vi "SDA - Analise e calibracao - COM CALC DE FREQ.vi"() -> ()   [LabVIEW 2019]
uses:
  <vilib>/Utility/file.llb/Read From Spreadsheet File (DBL).vi
  <vilib>/Utility/file.llb/Read Delimited Spreadsheet (DBL).vi
  <vilib>/Analysis/NI_AALPro.lvlib
  <vilib>/gmath/NI_Gmath.lvlib
  <vilib>/measure/NI_MABase.lvlib
panel:
  out "ROCOF deviation 2":dbl[](graph)
  in  "F/s":dbl=25.0 format="%#_13g"
  in  "upper":dbl=5.0 format="%#_13g"
  in  "bottom":dbl format="%#_13g"
  in  "bottom":i32=2
  in  "upper":i32=100
  in  "bottom":i32=2
  in  "upper":i32=50
  in  "K (%)":dbl=100.0 format="%#_13g"
  in  "bottom":i32=-180
  in  "upper":i32=180
  in  "upper":i32=65
  in  "bottom":i32=55
  in  "Amplitude base":dbl=1.25 format="%#_13g"
  in  "p.u. ?":bool=TRUE
  in  "Numeric":dbl
  out "output cluster":cluster{i32, i32}
  in  "offset":dbl format="%0.2p"
  in  "phase":dbl format="%.2p"
  in  "amplitude":dbl=1.0 format="%0.2p"
  in  "frequency":dbl=10.0 format="%0.2p"
  out "delay time":dbl format="%#_6f"
  in  "y":dbl
  out "fractional index or x":dbl format="%#_7g"
  in  "threshold y":dbl=0.95
  out "spread value":dbl
  out "lenght":i32
  in  "kept interval":i32=25
  out "Table 2":string[][](table)
  in  "Labels Size":u32=24
  in  "X label":T1(ring)=enum."medidas"
  in  "Tab Control":T2(tab)
  in  "Tab Control 2":T3(tab)
  out "Magnitude absolute deviation":dbl[](graph)
  out "Absolute phase deviation":dbl[](graph)
  out "Magnitude deviation":dbl[](graph)
  out "Phase deviation":dbl[](graph)
  out "Phase":dbl[][](graph)
  out "Magnitude":dbl[][](graph)
  out "TVE":dbl[](graph)
  in  "Tab Control 3":T3(tab)
  out "Absolute freq. deviation":dbl[](graph)
  out "Absolute ROCOF deviation":dbl[](graph)
  out "Frequency deviation":dbl[](graph)
  out "ROCOF deviation":dbl[](graph)
  out "Frequency":dbl[][](graph)
  out "ROCOF":dbl[][](graph)
  out "Frequency deviation 2":dbl[](graph)
  out "Curve fit":dbl[][](graph)
  out "ROCOF\nreference":dbl[](array[numeric])
  out "ROCOF\nmeasured":dbl[](array[numeric])
  out "Frequency\nmeasured":dbl[](array[numeric])
  out "Frequency\nreference":dbl[](array[numeric])
  out "Phase\nmeasured":dbl[](array[numeric])
  out "Phase\nreference":dbl[](array[numeric])
  out "Magnitude\nmeasured":dbl[](array[numeric])
  out "Magnitude\nreference":dbl[](array[numeric])
  in  "polynomial order":i32=2
  in  "Type":T4(ring)=enum."Linear"
  out "Coefficients":string[][](table) caption="Table"
  in  "X data":T5(ring)
  in  "Y data":T5(ring)=enum."Magnitude deviation"
  out "Fit deviation":dbl[](graph)
  out "Correlation\ncoefficient (R)":dbl format="%.7g"
  out "R^2":dbl format="%.7g"
  in  "busca freq":dbl
  out "XY Graph 3":cluster{dbl[], dbl[]}(graph)
  out "XY Graph 2":cluster{dbl[], dbl[]}(graph)
  out "fractional index":dbl format="%_6g"
  out "x*y":dbl
  in  "fractional index or x 3":dbl
  out "ângulo corresp":dbl
  out "mag correspondente":dbl
  in  "frequency 2":dbl
  out "TVE Histogram":T6(graph)
  out "Frequency Error Histogram":T6(graph)
  out "Magnitude Error Histogram":T6(graph)
  out "Phase Error Histogram":T6(graph)
  in  "final":i32
  in  "Interval":bool
  in  "index":i32
  out "nº de amostras":i32
  in  "del interval":i32=25
  in  "Exclude\ninterval":bool
  in  "Archive name":path=path "D:/Resultados/teste.txt"
  # "Fase x freq"
  # "Mag. x mag."
  # "Synchrophasors Data Analysis"
  # "Main Errors"
  # "Max"
  # "Mean"
  # "Min"
  # "Magnitude (%)"
  # "Phase (º)"
  # "TVE (%)"
  # "Freq. (Hz)"
  # "ROCOF (Hz/s)"
  # "Amplitude"
  # "Frequency"
  # "Phase"
  # "Harmonic"
  # "Freq. Interf."
  # "Modulation\nFrequency"
  # "Time"
  # "(frames/second)"
  # "Tamanho para dissertação:\n312x732"
  # "EXTRA"
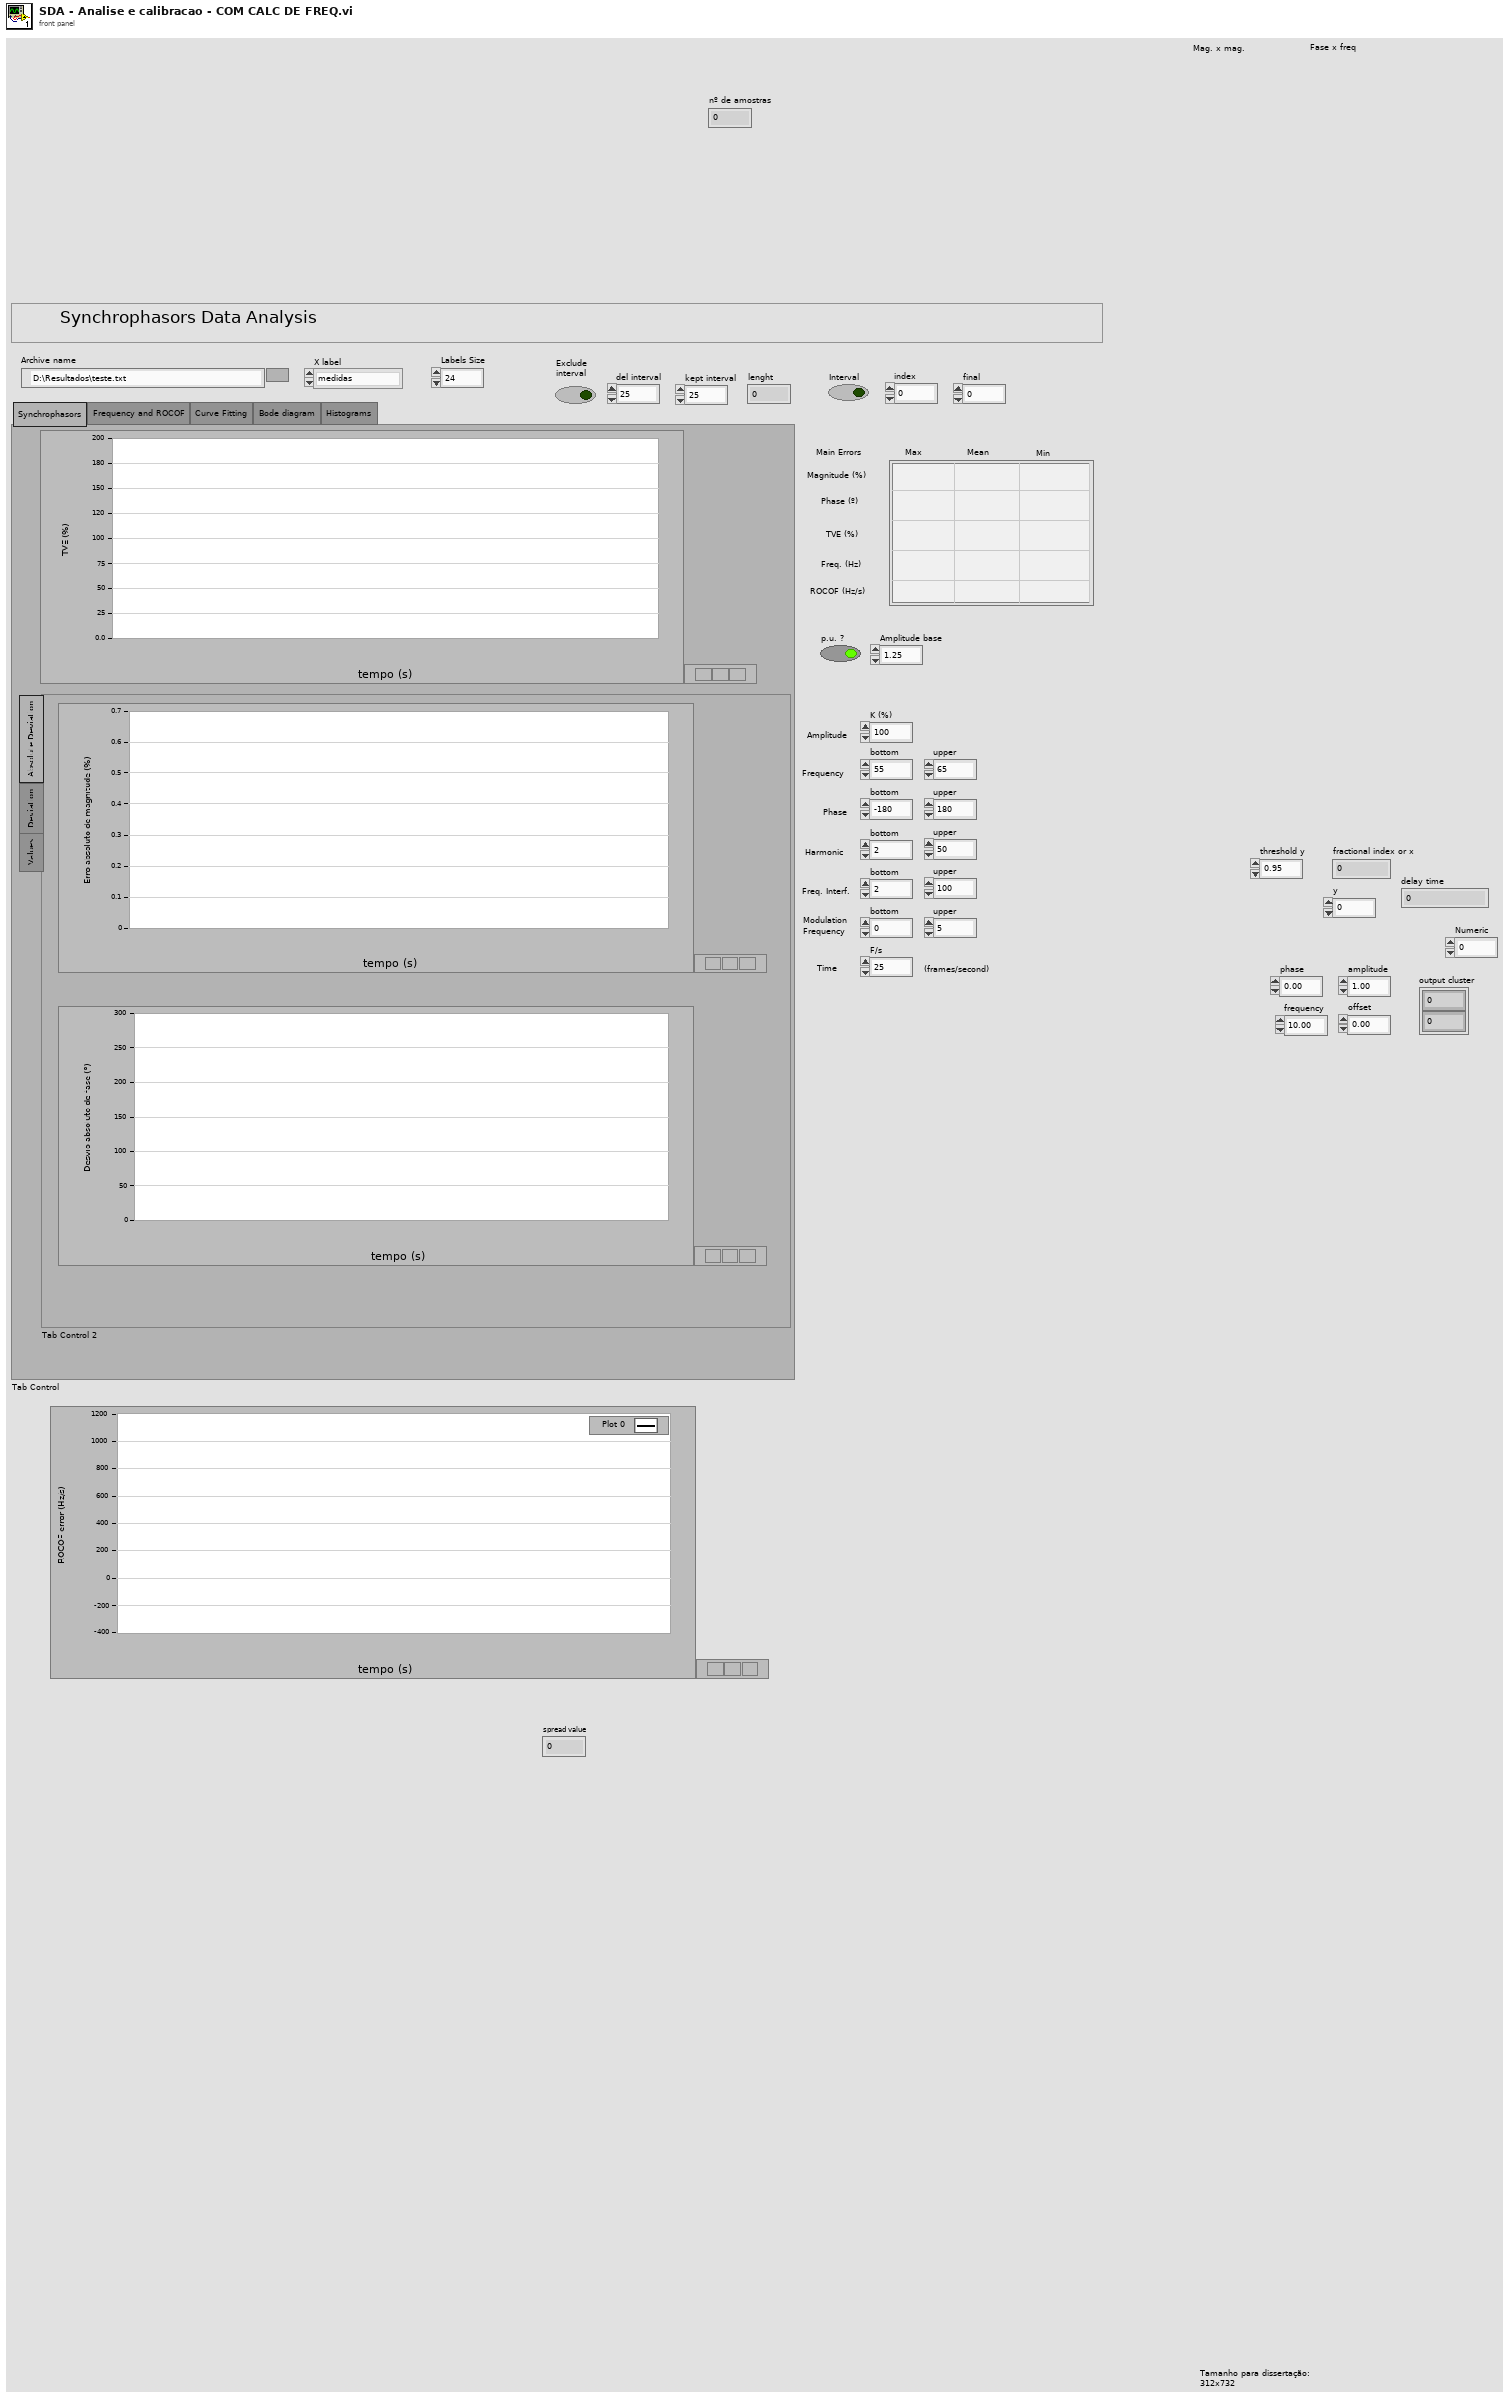
[diagram p1: front panel]
types:
  T1 = enum16{"tempo (s)", "medidas", "Amplitude (%)", "Ângulo (°)", "Frequência (Hz)", "ROCOF (Hz/s)", "Harmônica (.ª)", "Frequência de interferência (Hz)", "Frequência de modulação (Hz)"}
  T2 = enum32{"Synchrophasors", "Frequency and ROCOF", "Curve Fitting", "Bode diagram", "Histograms"}
  T3 = enum32{"Absolute Deviation", "Deviation", "Values"}
  T4 = enum16{"Exponencial", "Logarithm", "Linear", "Polynomial", "Sinusoidal"}
  T5 = enum16{"Magnitude reference", "Magnitude measured", "Magnitude deviation", "Phase reference", "Phase measured", "Phase deviation", "Frequency reference", "Frequency measured", "Frequency deviation"}
  T6 = cluster{"X Values":dbl[], "Histogram: h(x)":i32[]}
  T7 = cluster{"max ref":dbl, "min ref":dbl, "mean ref":dbl, "max dev":dbl, "min dev":dbl, "mean dev":dbl, "max meas":dbl, "min meas":dbl, "mean meas":dbl}
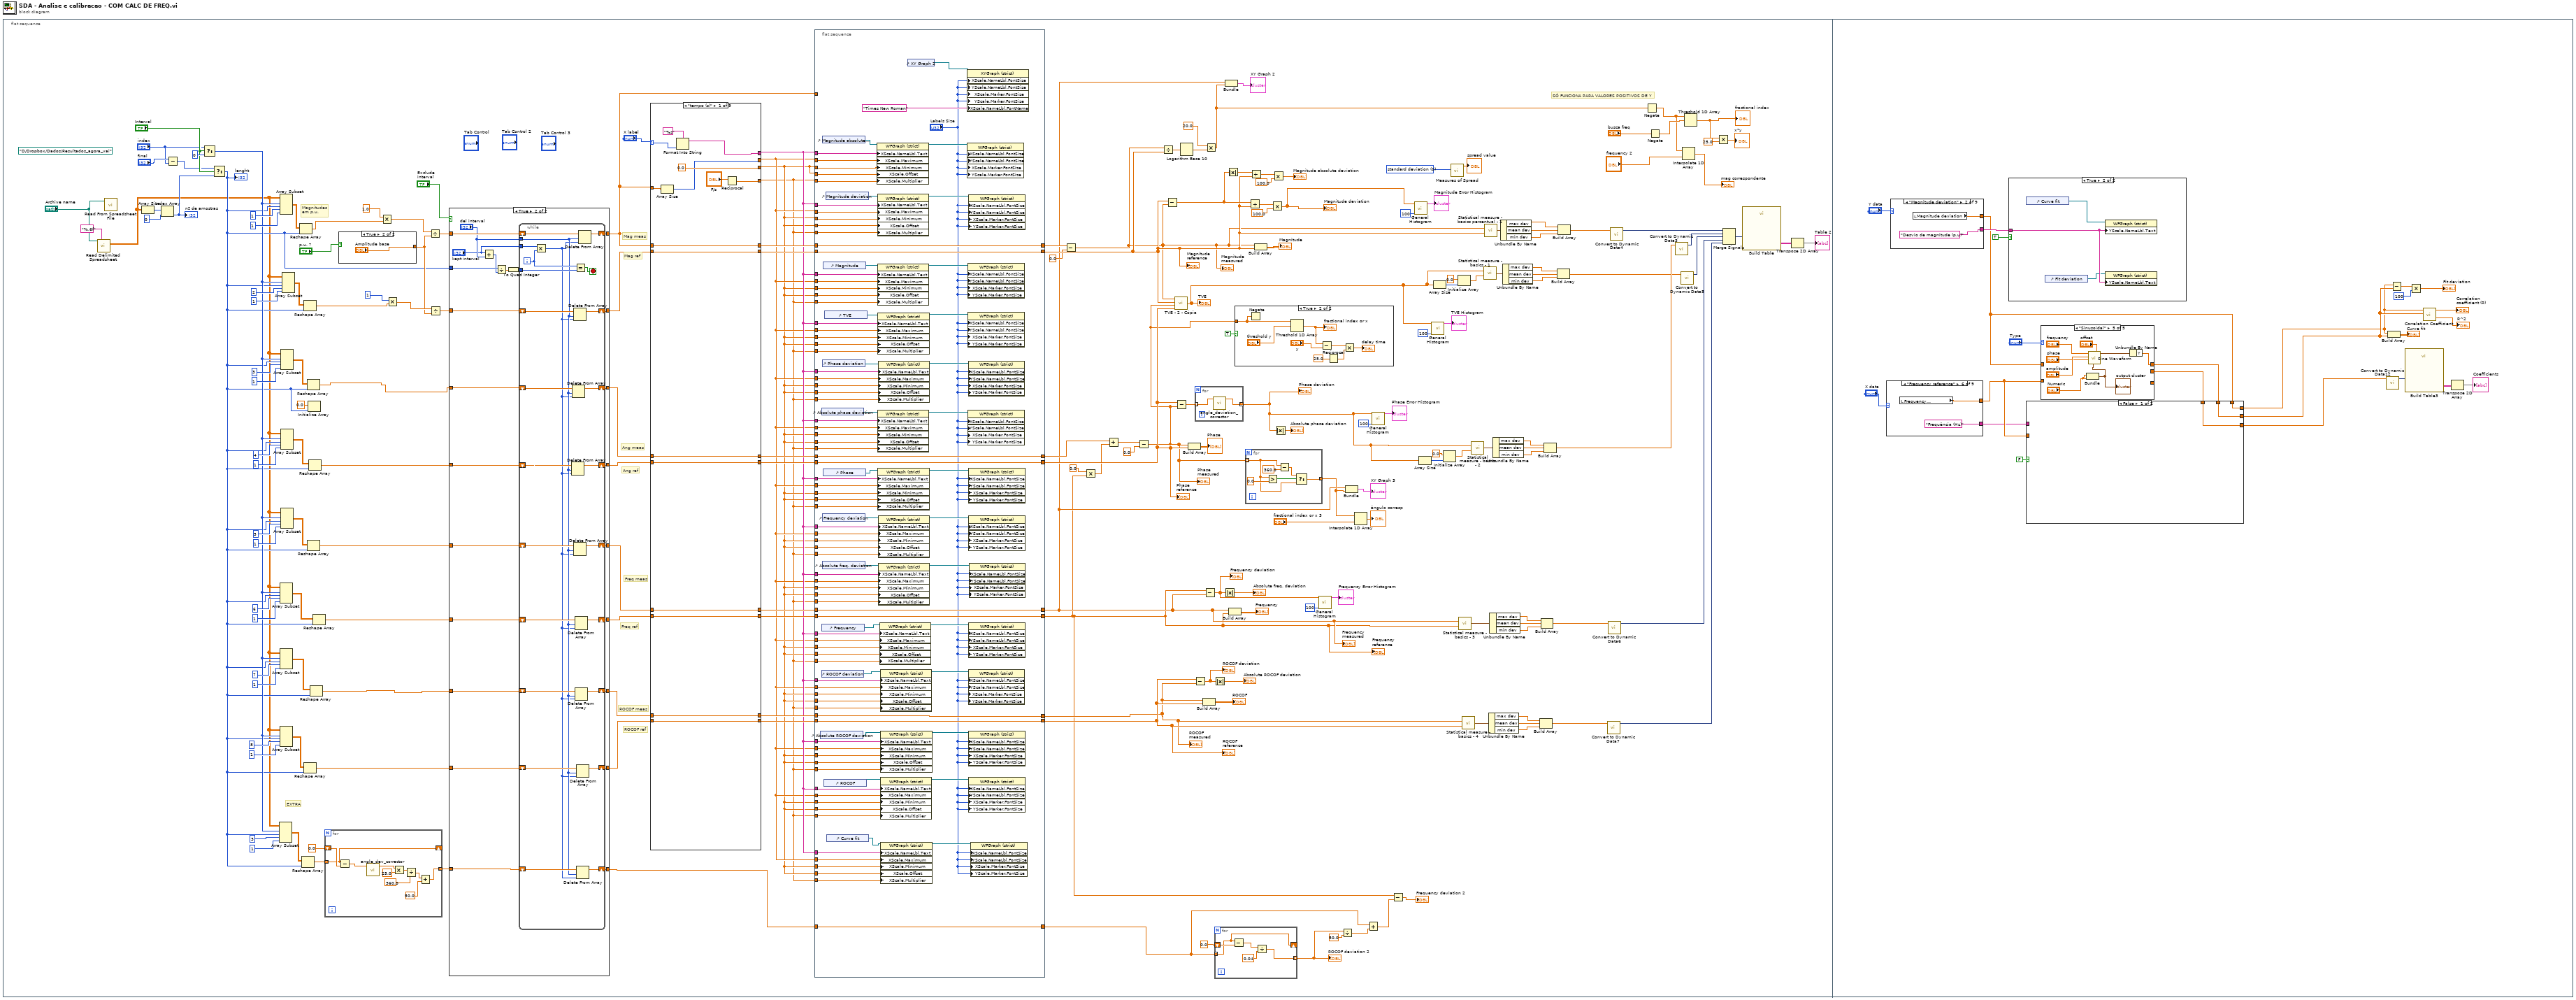
[diagram p0: block diagram]
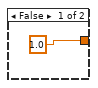
[diagram p3: hidden frame]
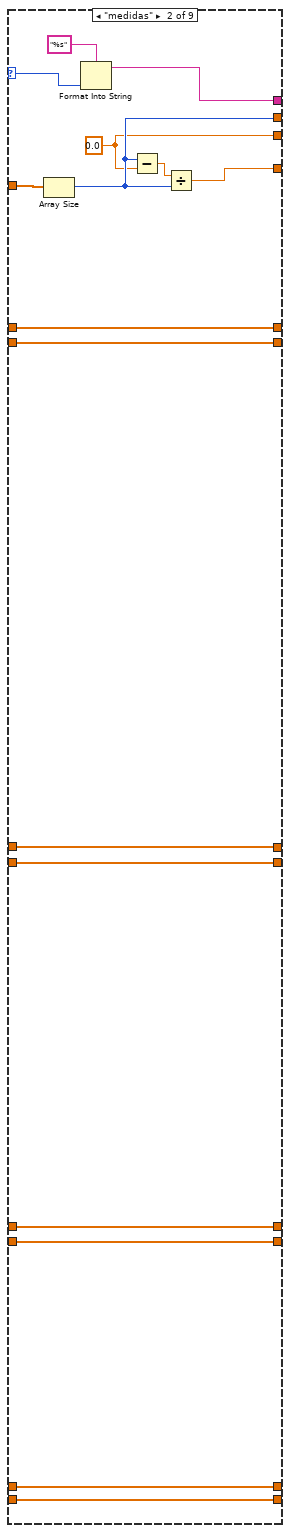
[diagram p4: hidden frame]
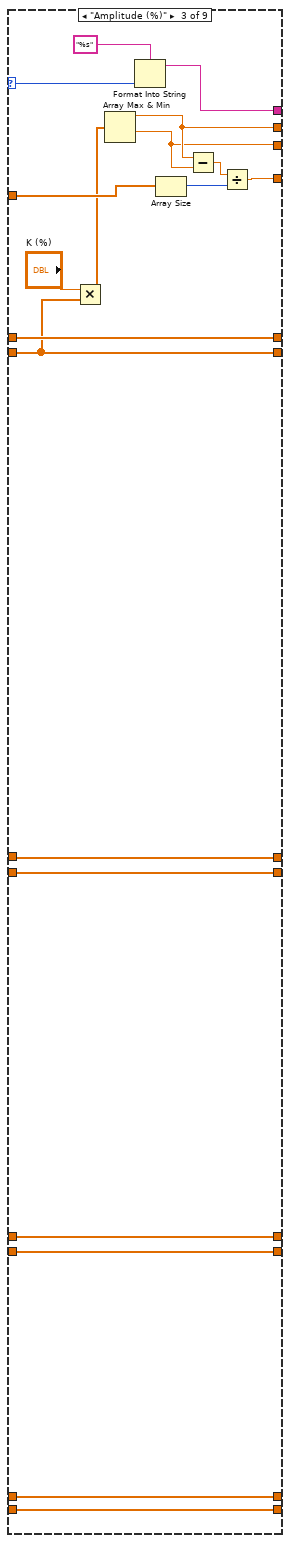
[diagram p5: hidden frame]
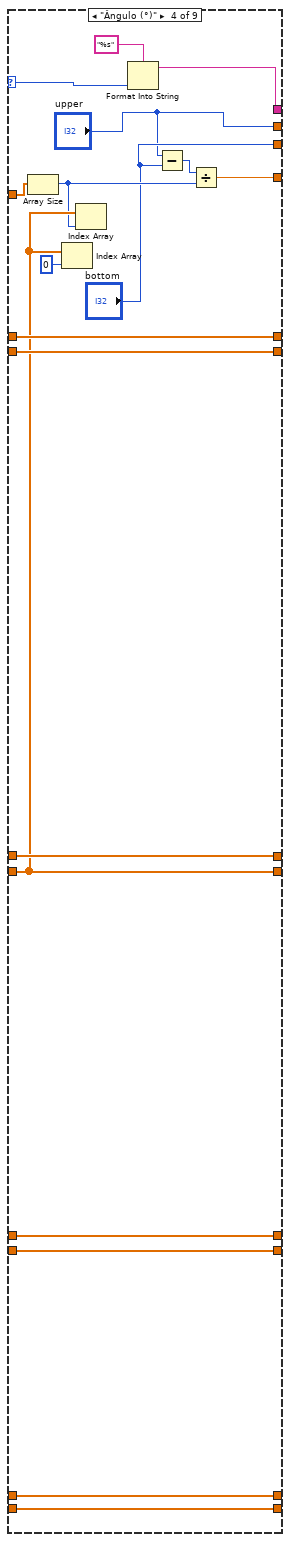
[diagram p6: hidden frame]
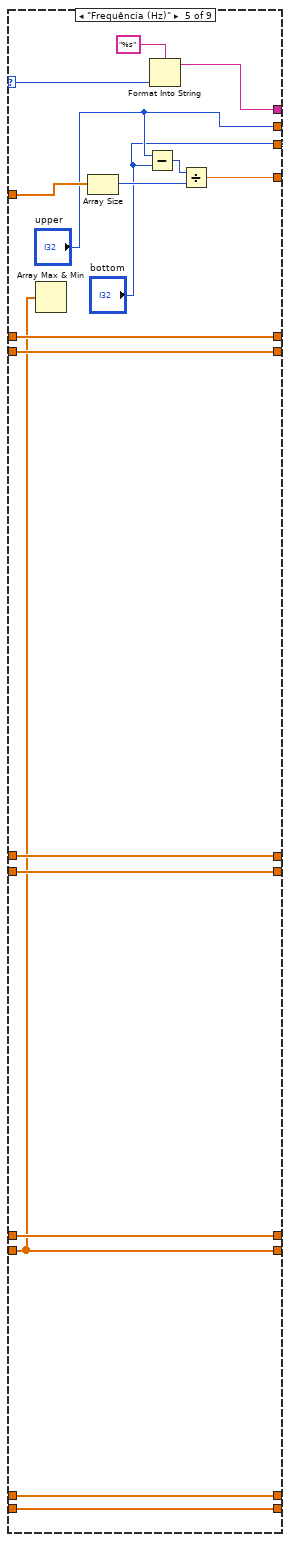
[diagram p7: hidden frame]
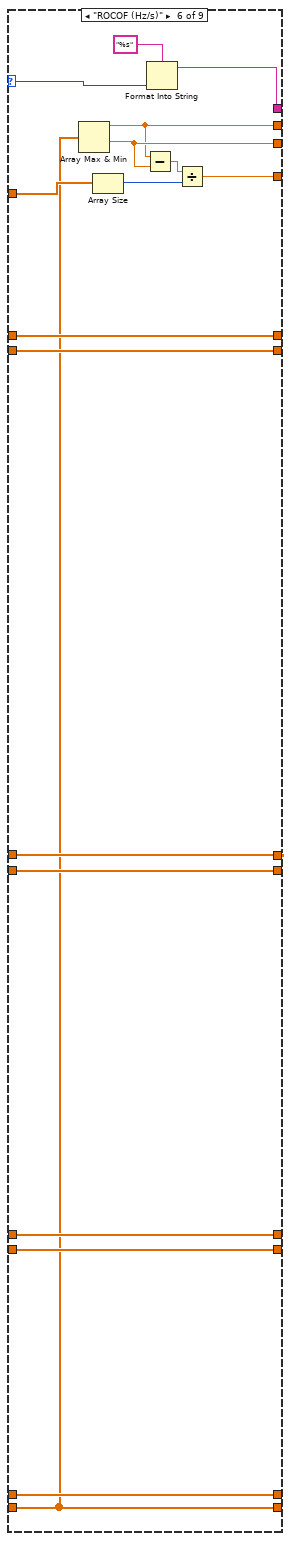
[diagram p8: hidden frame]
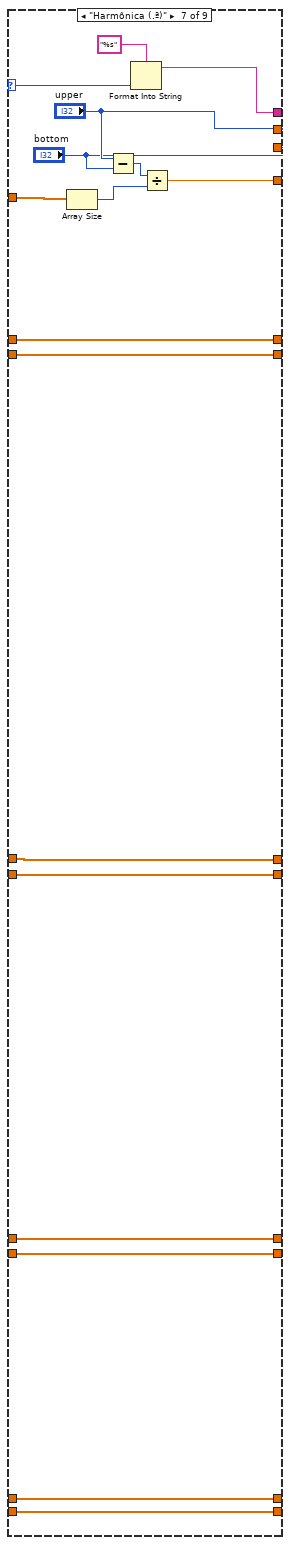
[diagram p9: hidden frame]
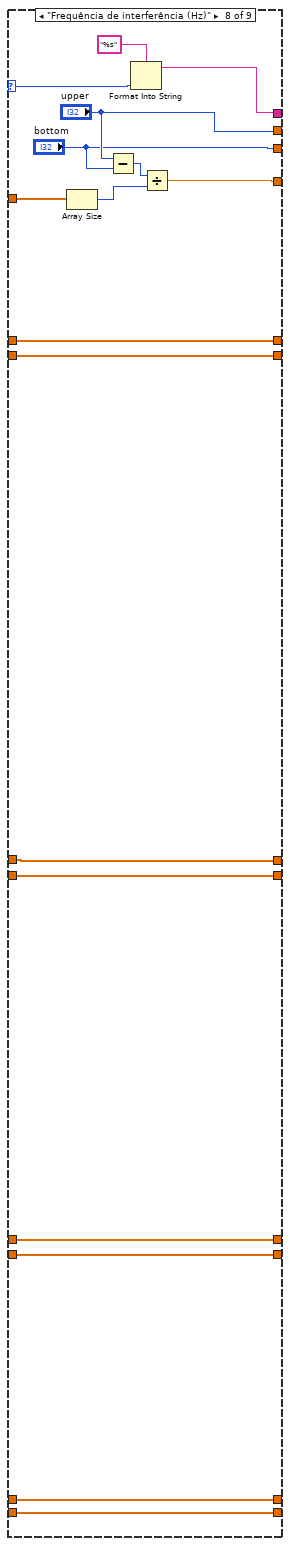
[diagram p10: hidden frame]
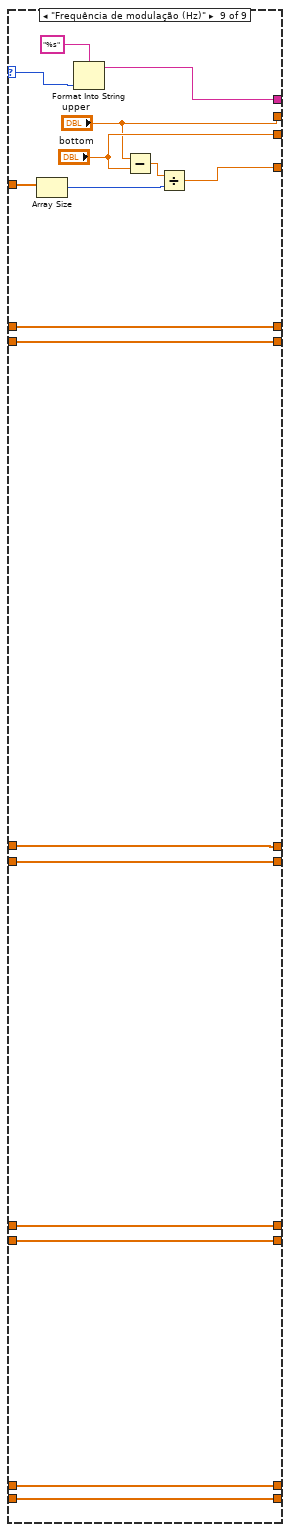
[diagram p11: hidden frame]
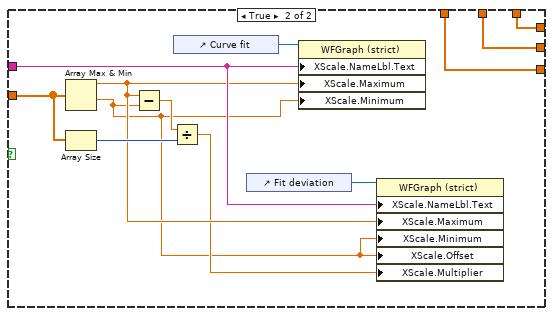
[diagram p13: hidden frame]
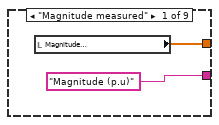
[diagram p15: hidden frame]
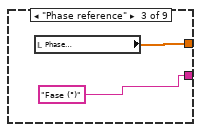
[diagram p16: hidden frame]
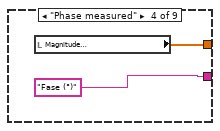
[diagram p17: hidden frame]
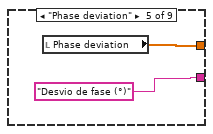
[diagram p18: hidden frame]
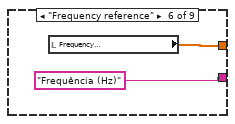
[diagram p19: hidden frame]
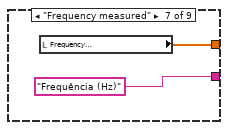
[diagram p20: hidden frame]
diagram:
  n1 = flat-sequence {
    frame #0 {
      w77 = 0 items=["standard deviation", "range", "mean absolute deviation", "interquartile range"] ("type")
      (unwired) path "D:/Dropbox/Dados/Resultados_agora_vai" ("file path (use dialog)")
      # "EXTRA"
      # "SÓ FUNCIONA PARA VALORES POSITIVOS DE Y"
      # "Magnitudes\nem p.u."
      # "ROCOF ref"
      # "ROCOF meas"
      # "Freq ref"
      # "Freq meas"
      # "Ang ref"
      # "Ang meas"
      # "Mag meas"
      # "Mag ref"
      n2 = call-poly <vilib>:"Read Delimited Spreadsheet.vi"("file path (dialog if empty)"="Archive name", "format (%.3f)"="%.6f") -> ("all rows"=w13:dbl[][])  [unwired: 8 in, 5 out]
      n3 = call-poly <vilib>:"Read From Spreadsheet File.vi"("file path (dialog if empty)"="Archive name") -> ()  [unwired: 6 in, 5 out]
      n4 = Array Size(array=w13) -> (size(s)=w189:i32[])
      n5 = Index Array(array=w189, index=0) -> (element=w121:i32)
      "nº de amostras" <- w121
      n6 = Subtract(x="final", y="index") -> (x-y=w124:i32)
      n7 = Select(t="index", s="Interval", f=0) -> (s? t:f=w17:i32)
      n8 = Select(t=w124, s="Interval", f=w121) -> (s? t:f=w16:i32)
      "lenght" <- w16
      n9 = Array Subset(array=w13, index (row)=w17, length (row)=w16, index (col)=3 ("index"), length (col)=1 ("length")) -> (w18:dbl[][])
      n10 = Array Subset(array=w13, index (row)=w17, length (row)=w16, index (col)=1 ("index"), length (col)=1 ("length")) -> (w190:dbl[][])
      n11 = Array Subset(array=w13, index (row)=w17, length (row)=w16, index (col)=6 ("index"), length (col)=1 ("length")) -> (w173:dbl[][])
      n12 = Array Subset(array=w13, index (row)=w17, length (row)=w16, index (col)=7 ("index"), length (col)=1 ("length")) -> (w170:dbl[][])
      n13 = Array Subset(array=w13, index (row)=w17, length (row)=w16, index (col)=8 ("index"), length (col)=1 ("length")) -> (w91:dbl[][])
      n14 = Array Subset(array=w13, index (row)=w17, length (row)=w16, index (col)=4 ("index"), length (col)=1 ("length")) -> (w179:dbl[][])
      n15 = Array Subset(array=w13, index (row)=w17, length (row)=w16, index (col)=5 ("index"), length (col)=1 ("length")) -> (w176:dbl[][])
      n16 = Array Subset(array=w13, index (row)=w17, length (row)=w16, index (col)=3 ("index"), length (col)=1 ("length")) -> (w182:dbl[][])
      n17 = Array Subset(array=w13, index (row)=w17, length (row)=w16, index (col)=2 ("index"), length (col)=1 ("length")) -> (w185:dbl[][])
      n18 = Reshape Array(w190, w16) -> (w69:dbl[])
      n19 = Reshape Array(w18, w16) -> (w8:dbl[])
      n20 = Reshape Array(w185, w16) -> (w67:dbl[])
      n21 = Reshape Array(w91, w16) -> (w90:dbl[])
      n22 = Reshape Array(w182, w16) -> (w39:dbl[])
      n23 = Reshape Array(w176, w16) -> (w142:dbl[])
      n24 = Initialize Array(0.0 ("element"), w16) -> ()  [unwired: 1 out]
      n25 = Reshape Array(w179, w16) -> (w141:dbl[])
      n26 = Reshape Array(w170, w16) -> (w23:dbl[])
      n27 = Reshape Array(w173, w16) -> (w143:dbl[])
      n28 = for {
        tunnel: w8 -> [w203] mode=indexing
        shift-right: [w203] -> _
        shift-left: 0.0 -> [w207]
        tunnel: [w201] -> w10 mode=indexing
        n29 = Subtract(x=w203, y=w207) -> (x-y=w199:dbl)
        n30 = call "angle_dev_corrector.vi"("angle"=w199) -> ("angle corrected"=w198:dbl)  [unwired: 6 in, 2 out]
        n31 = Multiply(x=w198, y=25.0) -> (x*y=w205:dbl)
        n32 = Divide(x=w205, y=360.0) -> (x/y=w200:dbl)
        n33 = Add(x=w200, y=50.0) -> (x+y=w201:dbl)
      }
      n34 = case shown="True" "p.u. ?" {
        tunnel: [1.0 "Amplitude base"] -> w22
        frame False {
        }
        frame True {
        }
      }
      n35 = Multiply(x=1.0, y=w69) -> (x*y=w68:dbl[])
      n36 = Multiply(x=1, y=w67) -> (x*y=w66:dbl[])
      n37 = Divide(x=w68, y=w22) -> (x/y=w101:dbl[])
      n38 = Divide(x=w66, y=w22) -> (x/y=w100:dbl[])
      n39 = case shown="True" "Exclude\ninterval" {
        tunnel: w101 -> [w498 w522]
        tunnel: [w498 w521] -> w58
        tunnel: w90 -> [w491 w517]
        tunnel: w23 -> [w492 w503]
        tunnel: w143 -> [w493 w514]
        tunnel: w142 -> [w494 w512]
        tunnel: w141 -> [w495 w510]
        tunnel: w39 -> [w496 w518]
        tunnel: w100 -> [w497 w520]
        tunnel: [w497 w519] -> w119
        tunnel: [w496 w508] -> w117
        tunnel: [w495 w509] -> w118
        tunnel: [w494 w511] -> w116
        tunnel: [w493 w513] -> w115
        tunnel: [w492 w515] -> w113
        tunnel: [w491 w516] -> w114
        tunnel: w16 -> [_ w507]
        tunnel: w10 -> [w490 w500]
        tunnel: [w490 w499] -> w9
        frame False {
        }
        frame True {
          n40 = Add(x="kept interval", y="del interval") -> (x+y=w505:i32)
          n41 = Divide(x=w507, y=w505) -> (x/y=w502:dbl)
          n42 = To Quad Integer(1:w502) -> (0:w501:i64)
          n43 = while {
            tunnel: "del interval" -> [w525]
            shift-right: [w544] -> w521
            shift-left: w522 -> [w545]
            shift-right: [w543] -> w519
            shift-left: w520 -> [w542]
            shift-right: [w540] -> w508
            shift-left: w518 -> [w541]
            shift-right: [w538] -> w509
            shift-left: w510 -> [w539]
            shift-right: [w536] -> w511
            shift-left: w512 -> [w537]
            shift-right: [w534] -> w513
            shift-left: w514 -> [w535]
            shift-right: [w532] -> w515
            shift-left: w503 -> [w533]
            shift-right: [w530] -> w516
            shift-left: w517 -> [w531]
            tunnel: w501 -> [w529]
            tunnel: "kept interval" -> [w527]
            shift-right: [w523] -> w499
            shift-left: w500 -> [w526]
            i -> [w528]
            stop <- w546 stop-if-true
            n44 = Multiply(x=w527, y=w528) -> (x*y=w524:i32)
            n45 = Delete From Array(array=w539, length=w525, index=w524) -> (array with subset deleted=w538:dbl[])  [unwired: 1 out]
            n46 = Delete From Array(array=w541, length=w525, index=w524) -> (array with subset deleted=w540:dbl[])  [unwired: 1 out]
            n47 = Delete From Array(array=w542, length=w525, index=w524) -> (array with subset deleted=w543:dbl[])  [unwired: 1 out]
            n48 = Delete From Array(array=w537, length=w525, index=w524) -> (array with subset deleted=w536:dbl[])  [unwired: 1 out]
            n49 = Equal?(x=w528, y=w529) -> (x = y?=w546:bool)
            n50 = Delete From Array(array=w535, length=w525, index=w524) -> (array with subset deleted=w534:dbl[])  [unwired: 1 out]
            n51 = Delete From Array(array=w533, length=w525, index=w524) -> (array with subset deleted=w532:dbl[])  [unwired: 1 out]
            n52 = Delete From Array(array=w531, length=w525, index=w524) -> (array with subset deleted=w530:dbl[])  [unwired: 1 out]
            n53 = Delete From Array(array=w526, length=w525, index=w524) -> (array with subset deleted=w523:dbl[])  [unwired: 1 out]
            n54 = Delete From Array(array=w545, length=w525, index=w524) -> (array with subset deleted=w544:dbl[])  [unwired: 1 out]
          }
        }
      }
      n55 = case shown="\"tempo (s)\"" "X label" {
        selector: "X label" -> [w341 w356 w375 w395 w411 w429 w454 w463 w482]
        tunnel: w58 -> [w342 w357 w386 w394 w412 w430 w451 w460 w483]
        tunnel: w119 -> [w350 w366 w372 w403 w409 w427 w448 w471 w485]
        tunnel: [w350 w366 w372 w403 w409 w427 w448 w471 w485] -> w103
        tunnel: w58 -> [w351 w367 w383 w404 w421 w428 w449 w472 w486]
        tunnel: [w351 w367 w383 w404 w421 w428 w449 w472 w486] -> w102
        tunnel: w118 -> [w348 w364 w381 w391 w419 w437 w447 w470 w477]
        tunnel: w117 -> [w349 w365 w382 w402 w420 w438 w439 w456 w478]
        tunnel: [w349 w365 w382 w402 w420 w438 w439 w456 w478] -> w104
        tunnel: [w348 w364 w381 w391 w419 w437 w447 w470 w477] -> w105
        tunnel: w116 -> [w347 w363 w380 w401 w418 w436 w446 w469 w476]
        tunnel: w115 -> [w346 w362 w379 w400 w408 w435 w445 w468 w475]
        tunnel: [w347 w363 w380 w401 w418 w436 w446 w469 w476] -> w107
        tunnel: [w346 w362 w379 w400 w408 w435 w445 w468 w475] -> w106
        tunnel: w114 -> [w344 w360 w378 w398 w416 w424 w443 w466 w473]
        tunnel: [w344 w360 w378 w398 w416 w424 w443 w466 w473] -> w109
        tunnel: w113 -> [w345 w361 w377 w399 w417 w434 w444 w467 w474]
        tunnel: [w345 w361 w377 w399 w417 w434 w444 w467 w474] -> w108
        tunnel: [w340 w355 w374 w393 w410 w426 w450 w464 w487] -> w74
        tunnel: [w338 w354 w370 "upper" "upper" w423 "upper" "upper" "upper"] -> w73
        tunnel: [0.0 ("X Scale.Offset and Multiplier:Offset") w353 w369 "bottom" "bottom" w425 "bottom" "bottom" "bottom"] -> w72
        tunnel: [w336 w352 w368 w389 w407 w422 w440 w457 w484] -> w71
        frame "tempo (s)" {
          n56 = Array Size(array=w342) -> (size(s)=w338:i32)
          n57 = Format Into String(format string="%s", w341) -> (resulting string=w340:string)  [unwired: 2 in, 1 out]
          n58 = Reciprocal(x="F/s") -> (1/x=w336:dbl)
        }
        frame "medidas" {
          w353 = 0.0 ("X Scale.Offset and Multiplier:Offset")
          n59 = Array Size(array=w357) -> (size(s)=w354:i32)
          n60 = Format Into String(format string="%s", w356) -> (resulting string=w355:string)  [unwired: 2 in, 1 out]
          n61 = Subtract(x=w354, y=w353) -> (x-y=w359:dbl)
          n62 = Divide(x=w359, y=w354) -> (x/y=w352:dbl)
        }
        frame "Amplitude (%)" {
          n63 = Multiply(x="K (%)", y=w372) -> (x*y=w371:dbl[])
          n64 = Array Max & Min(array=w371) -> (max value=w370:dbl, min value=w369:dbl)  [unwired: 2 out]
          n65 = Format Into String(format string="%s", w375) -> (resulting string=w374:string)  [unwired: 2 in, 1 out]
          n66 = Array Size(array=w386) -> (size(s)=w385:i32)
          n67 = Subtract(x=w370, y=w369) -> (x-y=w384:dbl)
          n68 = Divide(x=w384, y=w385) -> (x/y=w368:dbl)
        }
        frame "Ângulo (°)" {
          n69 = Array Size(array=w394) -> (size(s)=w390:i32)
          n70 = Index Array(array=w391, index=0) -> ()  [unwired: 1 out]
          n71 = Index Array(array=w391, index=w390) -> ()  [unwired: 1 out]
          n72 = Format Into String(format string="%s", w395) -> (resulting string=w393:string)  [unwired: 2 in, 1 out]
          n73 = Subtract(x="upper", y="bottom") -> (x-y=w397:i32)
          n74 = Divide(x=w397, y=w390) -> (x/y=w389:dbl)
        }
        frame "Frequência (Hz)" {
          n75 = Array Max & Min(array=w408) -> ()  [unwired: 4 out]
          n76 = Array Size(array=w412) -> (size(s)=w415:i32)
          n77 = Subtract(x="upper", y="bottom") -> (x-y=w414:i32)
          n78 = Format Into String(format string="%s", w411) -> (resulting string=w410:string)  [unwired: 2 in, 1 out]
          n79 = Divide(x=w414, y=w415) -> (x/y=w407:dbl)
        }
        frame "ROCOF (Hz/s)" {
          n80 = Array Max & Min(array=w424) -> (max value=w423:dbl, min value=w425:dbl)  [unwired: 2 out]
          n81 = Array Size(array=w430) -> (size(s)=w433:i32)
          n82 = Subtract(x=w423, y=w425) -> (x-y=w432:dbl)
          n83 = Format Into String(format string="%s", w429) -> (resulting string=w426:string)  [unwired: 2 in, 1 out]
          n84 = Divide(x=w432, y=w433) -> (x/y=w422:dbl)
        }
        frame "Harmônica (.ª)" {
          n85 = Array Size(array=w451) -> (size(s)=w453:i32)
          n86 = Subtract(x="upper", y="bottom") -> (x-y=w452:i32)
          n87 = Format Into String(format string="%s", w454) -> (resulting string=w450:string)  [unwired: 2 in, 1 out]
          n88 = Divide(x=w452, y=w453) -> (x/y=w440:dbl)
        }
        frame "Frequência de interferência (Hz)" {
          n89 = Array Size(array=w460) -> (size(s)=w462:i32)
          n90 = Subtract(x="upper", y="bottom") -> (x-y=w461:i32)
          n91 = Format Into String(format string="%s", w463) -> (resulting string=w464:string)  [unwired: 2 in, 1 out]
          n92 = Divide(x=w461, y=w462) -> (x/y=w457:dbl)
        }
        frame "Frequência de modulação (Hz)" {
          n93 = Array Size(array=w483) -> (size(s)=w481:i32)
          n94 = Format Into String(format string="%s", w482) -> (resulting string=w487:string)  [unwired: 2 in, 1 out]
          n95 = Subtract(x="upper", y="bottom") -> (x-y=w489:dbl)
          n96 = Divide(x=w489, y=w481) -> (x/y=w484:dbl)
        }
      }
      n97 = flat-sequence {
        tunnel: w74 -> [w335]
        tunnel: w74 -> [w334]
        tunnel: w74 -> [w333]
        tunnel: w73 -> [w332]
        tunnel: w72 -> [w331]
        tunnel: w72 -> [w330]
        tunnel: w71 -> [w329]
        tunnel: w73 -> [w328]
        tunnel: w72 -> [w327]
        tunnel: w72 -> [w326]
        tunnel: w71 -> [w325]
        tunnel: w74 -> [w324]
        tunnel: w74 -> [w323]
        tunnel: w74 -> [w322]
        tunnel: w71 -> [w321]
        tunnel: w72 -> [w320]
        tunnel: w72 -> [w319]
        tunnel: w73 -> [w318]
        tunnel: w71 -> [w317]
        tunnel: w72 -> [w316]
        tunnel: w72 -> [w315]
        tunnel: w73 -> [w314]
        tunnel: w74 -> [w313]
        tunnel: w71 -> [w312]
        tunnel: w72 -> [w311]
        tunnel: w72 -> [w310]
        tunnel: w73 -> [w309]
        tunnel: w73 -> [w308]
        tunnel: w72 -> [w307]
        tunnel: w72 -> [w306]
        tunnel: w71 -> [w305]
        tunnel: w73 -> [w304]
        tunnel: w72 -> [w303]
        tunnel: w72 -> [w302]
        tunnel: w71 -> [w301]
        tunnel: w74 -> [w300]
        tunnel: w74 -> [w299]
        tunnel: w73 -> [w298]
        tunnel: w72 -> [w297]
        tunnel: w72 -> [w296]
        tunnel: w71 -> [w295]
        tunnel: w74 -> [w294]
        tunnel: w73 -> [w293]
        tunnel: w72 -> [w292]
        tunnel: w72 -> [w291]
        tunnel: w71 -> [w290]
        tunnel: w74 -> [w289]
        tunnel: w73 -> [w288]
        tunnel: w72 -> [w287]
        tunnel: w72 -> [w286]
        tunnel: w71 -> [w285]
        tunnel: w74 -> [w284]
        tunnel: w73 -> [w283]
        tunnel: w72 -> [w282]
        tunnel: w72 -> [w281]
        tunnel: w71 -> [w280]
        tunnel: w74 -> [w279]
        tunnel: w73 -> [w278]
        tunnel: w72 -> [w277]
        tunnel: w72 -> [w276]
        tunnel: w71 -> [w275]
        tunnel: w71 -> [w274]
        tunnel: w72 -> [w273]
        tunnel: w72 -> [w272]
        tunnel: w73 -> [w271]
        tunnel: w109 -> [w244]
        tunnel: [w244] -> w62
        tunnel: [w243] -> w61
        tunnel: w108 -> [w243]
        tunnel: w107 -> [w242]
        tunnel: [w242] -> w21
        tunnel: w106 -> [w241]
        tunnel: [w241] -> w12
        tunnel: w105 -> [w240]
        tunnel: w104 -> [w239]
        tunnel: [w240] -> w78
        tunnel: [w239] -> w29
        tunnel: [w237] -> w31
        tunnel: [w238] -> w60
        tunnel: w103 -> [w238]
        tunnel: w102 -> [w237]
        tunnel: w74 -> [w234]
        tunnel: w73 -> [w233]
        tunnel: w72 -> [w232]
        tunnel: w72 -> [w231]
        tunnel: w71 -> [w230]
        tunnel: w58 -> [_]
        tunnel: w9 -> [w226]
        tunnel: [w226] -> w3
        frame #0 {
          n98 = control-ref of="Absolute ROCOF deviation"() -> (w254:refnum<vi>)
          n99 = control-ref of="Absolute phase deviation"() -> (w261:refnum<vi>)
          n100 = control-ref of="ROCOF deviation"() -> (w255:refnum<vi>)
          n101 = control-ref of="Frequency"() -> (w256:refnum<vi>)
          n102 = control-ref of="Magnitude absolute deviation"() -> (w246:refnum<vi>)
          n103 = control-ref of="Phase deviation"() -> (w262:refnum<vi>)
          n104 = control-ref of="Absolute freq. deviation"() -> (w257:refnum<vi>)
          n105 = control-ref of="Frequency deviation"() -> (w258:refnum<vi>)
          n106 = control-ref of="Magnitude"() -> (w245:refnum<vi>)
          n107 = control-ref of="Phase"() -> (w260:refnum<vi>)
          n108 = control-ref of="ROCOF"() -> (w253:refnum<vi>)
          n109 = control-ref of="TVE"() -> (w263:refnum<vi>)
          n110 = control-ref of="Magnitude deviation"() -> (w269:refnum<vi>)
          n111 = control-ref of="Curve fit"() -> (w235:refnum<vi>)
          n112 = property on="Property Node" class="WFGraph (strict)"(reference=w246, "XScale.NameLbl.Text"=w335, "XScale.Maximum"=w332, "XScale.Minimum"=w331, "XScale.Offset"=w330, "XScale.Multiplier"=w329) -> (reference out=w270:refnum<vi>)  [unwired: 1 in, 1 out]
          n113 = property on="Property Node" class="WFGraph (strict)"(reference=w269, "XScale.NameLbl.Text"=w334, "XScale.Maximum"=w328, "XScale.Minimum"=w327, "XScale.Offset"=w326, "XScale.Multiplier"=w325) -> (reference out=w268:refnum<vi>)  [unwired: 1 in, 1 out]
          n114 = property on="Property Node" class="WFGraph (strict)"(reference=w245, "XScale.NameLbl.Text"=w333, "XScale.Maximum"=w314, "XScale.Minimum"=w315, "XScale.Offset"=w316, "XScale.Multiplier"=w317) -> (reference out=w266:refnum<vi>)  [unwired: 1 in, 1 out]
          n115 = property on="Property Node" class="WFGraph (strict)"(reference=w261, "XScale.NameLbl.Text"=w324, "XScale.Maximum"=w304, "XScale.Minimum"=w303, "XScale.Offset"=w302, "XScale.Multiplier"=w301) -> (reference out=w264:refnum<vi>)  [unwired: 1 in, 1 out]
          n116 = property on="Property Node" class="WFGraph (strict)"(reference=w263, "XScale.NameLbl.Text"=w322, "XScale.Maximum"=w318, "XScale.Minimum"=w319, "XScale.Offset"=w320, "XScale.Multiplier"=w321) -> (reference out=w267:refnum<vi>)  [unwired: 1 in, 1 out]
          n117 = property on="Property Node" class="WFGraph (strict)"(reference=w260, "XScale.NameLbl.Text"=w313, "XScale.Maximum"=w309, "XScale.Minimum"=w310, "XScale.Offset"=w311, "XScale.Multiplier"=w312) -> (reference out=w259:refnum<vi>)  [unwired: 1 in, 1 out]
          n118 = property on="Property Node" class="WFGraph (strict)"(reference=w262, "XScale.NameLbl.Text"=w323, "XScale.Maximum"=w308, "XScale.Minimum"=w307, "XScale.Offset"=w306, "XScale.Multiplier"=w305) -> (reference out=w265:refnum<vi>)  [unwired: 1 in, 1 out]
          n119 = property on="Property Node" class="WFGraph (strict)"(reference=w258, "XScale.NameLbl.Text"=w300, "XScale.Maximum"=w271, "XScale.Minimum"=w272, "XScale.Offset"=w273, "XScale.Multiplier"=w274) -> (reference out=w252:refnum<vi>)  [unwired: 1 in, 1 out]
          n120 = property on="Property Node" class="WFGraph (strict)"(reference=w257, "XScale.NameLbl.Text"=w299, "XScale.Maximum"=w298, "XScale.Minimum"=w297, "XScale.Offset"=w296, "XScale.Multiplier"=w295) -> (reference out=w251:refnum<vi>)  [unwired: 1 in, 1 out]
          n121 = property on="Property Node" class="WFGraph (strict)"(reference=w256, "XScale.NameLbl.Text"=w294, "XScale.Maximum"=w293, "XScale.Minimum"=w292, "XScale.Offset"=w291, "XScale.Multiplier"=w290) -> (reference out=w250:refnum<vi>)  [unwired: 1 in, 1 out]
          n122 = property on="Property Node" class="WFGraph (strict)"(reference=w255, "XScale.NameLbl.Text"=w289, "XScale.Maximum"=w288, "XScale.Minimum"=w287, "XScale.Offset"=w286, "XScale.Multiplier"=w285) -> (reference out=w249:refnum<vi>)  [unwired: 1 in, 1 out]
          n123 = property on="Property Node" class="WFGraph (strict)"(reference=w253, "XScale.NameLbl.Text"=w279, "XScale.Maximum"=w278, "XScale.Minimum"=w277, "XScale.Offset"=w276, "XScale.Multiplier"=w275) -> (reference out=w247:refnum<vi>)  [unwired: 1 in, 1 out]
          n124 = property on="Property Node" class="WFGraph (strict)"(reference=w254, "XScale.NameLbl.Text"=w284, "XScale.Maximum"=w283, "XScale.Minimum"=w282, "XScale.Offset"=w281, "XScale.Multiplier"=w280) -> (reference out=w248:refnum<vi>)  [unwired: 1 in, 1 out]
          n125 = property on="Property Node" class="WFGraph (strict)"(reference=w235, "XScale.NameLbl.Text"=w234, "XScale.Maximum"=w233, "XScale.Minimum"=w232, "XScale.Offset"=w231, "XScale.Multiplier"=w230) -> (reference out=w236:refnum<vi>)  [unwired: 1 in, 1 out]
          n126 = control-ref of="XY Graph 2"() -> (w229:refnum<vi>)
          n127 = property class="XYGraph (strict)"(reference=w229, "XScale.NameLbl.FontSize"="Labels Size", "YScale.NameLbl.FontSize"="Labels Size", "XScale.Marker.FontSize"="Labels Size", "YScale.Marker.FontSize"="Labels Size", "XScale.NameLbl.FontName"="Times New Roman" ("X Scale.Name Label.Font:Name")) -> ()  [unwired: 1 in, 2 out]
          n128 = property class="WFGraph (strict)"(reference=w270, "XScale.NameLbl.FontSize"="Labels Size", "YScale.NameLbl.FontSize"="Labels Size", "XScale.Marker.FontSize"="Labels Size", "YScale.Marker.FontSize"="Labels Size") -> ()  [unwired: 1 in, 2 out]
          n129 = property class="WFGraph (strict)"(reference=w266, "XScale.NameLbl.FontSize"="Labels Size", "YScale.NameLbl.FontSize"="Labels Size", "XScale.Marker.FontSize"="Labels Size", "YScale.Marker.FontSize"="Labels Size") -> ()  [unwired: 1 in, 2 out]
          n130 = property class="WFGraph (strict)"(reference=w267, "XScale.NameLbl.FontSize"="Labels Size", "YScale.NameLbl.FontSize"="Labels Size", "XScale.Marker.FontSize"="Labels Size", "YScale.Marker.FontSize"="Labels Size") -> ()  [unwired: 1 in, 2 out]
          n131 = property class="WFGraph (strict)"(reference=w264, "XScale.NameLbl.FontSize"="Labels Size", "YScale.NameLbl.FontSize"="Labels Size", "XScale.Marker.FontSize"="Labels Size", "YScale.Marker.FontSize"="Labels Size") -> ()  [unwired: 1 in, 2 out]
          n132 = property class="WFGraph (strict)"(reference=w265, "XScale.NameLbl.FontSize"="Labels Size", "YScale.NameLbl.FontSize"="Labels Size", "XScale.Marker.FontSize"="Labels Size", "YScale.Marker.FontSize"="Labels Size") -> ()  [unwired: 1 in, 2 out]
          n133 = property class="WFGraph (strict)"(reference=w249, "XScale.NameLbl.FontSize"="Labels Size", "YScale.NameLbl.FontSize"="Labels Size", "XScale.Marker.FontSize"="Labels Size", "YScale.Marker.FontSize"="Labels Size") -> ()  [unwired: 1 in, 2 out]
          n134 = property class="WFGraph (strict)"(reference=w268, "XScale.NameLbl.FontSize"="Labels Size", "YScale.NameLbl.FontSize"="Labels Size", "XScale.Marker.FontSize"="Labels Size", "YScale.Marker.FontSize"="Labels Size") -> ()  [unwired: 1 in, 2 out]
          n135 = property class="WFGraph (strict)"(reference=w259, "XScale.NameLbl.FontSize"="Labels Size", "YScale.NameLbl.FontSize"="Labels Size", "XScale.Marker.FontSize"="Labels Size", "YScale.Marker.FontSize"="Labels Size") -> ()  [unwired: 1 in, 2 out]
          n136 = property class="WFGraph (strict)"(reference=w252, "XScale.NameLbl.FontSize"="Labels Size", "YScale.NameLbl.FontSize"="Labels Size", "XScale.Marker.FontSize"="Labels Size", "YScale.Marker.FontSize"="Labels Size") -> ()  [unwired: 1 in, 2 out]
          n137 = property class="WFGraph (strict)"(reference=w250, "XScale.NameLbl.FontSize"="Labels Size", "YScale.NameLbl.FontSize"="Labels Size", "XScale.Marker.FontSize"="Labels Size", "YScale.Marker.FontSize"="Labels Size") -> ()  [unwired: 1 in, 2 out]
          n138 = property class="WFGraph (strict)"(reference=w248, "XScale.NameLbl.FontSize"="Labels Size", "YScale.NameLbl.FontSize"="Labels Size", "XScale.Marker.FontSize"="Labels Size", "YScale.Marker.FontSize"="Labels Size") -> ()  [unwired: 1 in, 2 out]
          n139 = property class="WFGraph (strict)"(reference=w247, "XScale.NameLbl.FontSize"="Labels Size", "YScale.NameLbl.FontSize"="Labels Size", "XScale.Marker.FontSize"="Labels Size", "YScale.Marker.FontSize"="Labels Size") -> ()  [unwired: 1 in, 2 out]
          n140 = property class="WFGraph (strict)"(reference=w251, "XScale.NameLbl.FontSize"="Labels Size", "YScale.NameLbl.FontSize"="Labels Size", "XScale.Marker.FontSize"="Labels Size", "YScale.Marker.FontSize"="Labels Size") -> ()  [unwired: 1 in, 2 out]
          n141 = property class="WFGraph (strict)"(reference=w236, "XScale.NameLbl.FontSize"="Labels Size", "YScale.NameLbl.FontSize"="Labels Size", "XScale.Marker.FontSize"="Labels Size", "YScale.Marker.FontSize"="Labels Size") -> ()  [unwired: 1 in, 2 out]
        }
      }
      n142 = Subtract(x=w31, y=0.0 ("x")) -> (x-y=w30:dbl[])
      "Magnitude\nmeasured" <- w30
      n143 = Multiply(x=0.0, y=w12) -> (x*y=w28:dbl[])
      n144 = Add(x=w29, y=w28) -> (x+y=w25:dbl[])
      n145 = Subtract(x=w25, y=0.0 ("x")) -> (x-y=w26:dbl[])
      "Phase\nmeasured" <- w26
      n146 = Divide(x=w30, y=w60) -> (x/y=w55:dbl[])
      n147 = Subtract(x=w60, y=w30) -> (x-y=w128:dbl[])
      n148 = call "TVE - 2 - Cópia.vi"("Angle reference"=w78, "Angle measured"=w26, "Voltage reference"=w60, "Voltage measured"=w30) -> ("Array"=w38:dbl[])
      "TVE" <- w38
      n149 = Subtract(x=w78, y=w26) -> (x-y=w172:dbl[])
      n150 = Logarithm Base 10(1:w55) -> (0:w59:dbl[])
      n151 = Build Array(w26, w78) -> (→"Phase":dbl[][])
      n152 = Subtract(x=w62, y=w61) -> (x-y=w125:dbl[])
      "ROCOF deviation" <- w125
      n153 = for {
        tunnel: w172 -> [w224] mode=indexing
        tunnel: [w225] -> w34 mode=indexing
        n154 = call "angle_deviation_corrector.vi"("angle"=w224) -> ("angle corrected"=w225:dbl)  [unwired: 6 in, 2 out]
      }
      "Phase deviation" <- w34
      n155 = Build Array(w61, w62) -> (→"ROCOF":dbl[][])
      n156 = Subtract(x=w12, y=w21) -> (x-y=w37:dbl[])
      "Frequency deviation" <- w37
      n157 = Multiply(x=20.0, y=w59) -> (x*y=w49:dbl[])
      n158 = Absolute Value(x=w125) -> (abs(x)=→"Absolute ROCOF deviation":dbl[])
      n159 = for {
        tunnel: w3 -> [w194] mode=indexing
        shift-right: [w194] -> _
        shift-left: 0.0 -> [w197]
        tunnel: [w193] -> w6 mode=indexing
        n160 = Subtract(x=w194, y=w197) -> (x-y=w196:dbl)
        n161 = Divide(x=w196, y=0.04) -> (x/y=w193:dbl)
      }
      "ROCOF deviation 2" <- w6
      n162 = Absolute Value(x=w37) -> (abs(x)=→"Absolute freq. deviation":dbl[])
      n163 = Bundle(w21, w49) -> (→"XY Graph 2":cluster{dbl[], dbl[]})  [unwired: 1 in]
      n164 = Absolute Value(x=w128) -> (abs(x)=w132:dbl[])
      n165 = Build Array(w21, w12) -> (→"Frequency":dbl[][])
      n166 = case shown="True" TRUE {
        tunnel: w26 -> [_ w208]
        frame False {
        }
        frame True {
          n167 = Negate(x=w208) -> ()  [unwired: 1 out]
          n168 = Threshold 1D Array(2:"threshold y", 3:w208) -> (0:w215:dbl)  [unwired: 1 in]
          "fractional index or x" <- w215
          n169 = Subtract(x=w215, y="y") -> (x-y=w214:dbl)
          n170 = Reciprocal(x=25.0) -> (1/x=w212:dbl)
          n171 = Multiply(x=w214, y=w212) -> (x*y=→"delay time":dbl)
        }
      }
      n172 = for {
        tunnel: w26 -> [w218] mode=indexing
        tunnel: [w216] -> w46 mode=indexing
        n173 = Greater?(x=w218, y=0.0) -> (0:w220:bool)
        n174 = Subtract(x=w218, y=360.0) -> (x-y=w217:dbl)
        n175 = Select(t=w217, s=w220, f=w218) -> (s? t:f=w216:dbl)
      }
      n176 = Divide(x=w128, y=w60) -> (x/y=w130:dbl[])
      n177 = Divide(x=w132, y=w60) -> (x/y=w133:dbl[])
      n178 = Build Array(w30, w60) -> (→"Magnitude":dbl[][])
      n179 = Multiply(x=w130, y=100.0 ("x")) -> (x*y=w33:dbl[])
      "Magnitude deviation" <- w33
      n180 = Multiply(x=w133, y=100.0 ("x")) -> (x*y=→"Magnitude absolute deviation":dbl[])
      n181 = Absolute Value(x=w34) -> (abs(x)=→"Absolute phase deviation":dbl[])
      n182 = call <vilib>:"General Histogram.vi"("X"=w37, "# bins"=100) -> ("Histogram Graph"=→"Frequency Error Histogram":T6)  [unwired: 9 in, 4 out]
      n183 = Divide(x=w6, y=50.0) -> (x/y=w4:dbl[])
      n184 = Bundle(w21, w46) -> (→"XY Graph 3":cluster{dbl[], dbl[]})  [unwired: 1 in]
      n185 = Interpolate 1D Array(1:"fractional index or x 3", 2:w46) -> (0:→"ângulo corresp":dbl)
      n186 = Add(x=w3, y=w4) -> (x+y=w2:dbl[])
      n187 = call <vilib>:"General Histogram.vi"("X"=w34, "# bins"=100) -> ("Histogram Graph"=→"Phase Error Histogram":T6)  [unwired: 9 in, 4 out]
      n188 = Subtract(x=w12, y=w2) -> (x-y=→"Frequency deviation 2":dbl[])
      n189 = call <vilib>:"General Histogram.vi"("X"=w33, "# bins"=100) -> ("Histogram Graph"=→"Magnitude Error Histogram":T6)  [unwired: 9 in, 4 out]
      n190 = Array Size(array=w34) -> (size(s)=w137:i32)
      n191 = call <vilib>:"General Histogram.vi"("X"=w38, "# bins"=100) -> ("Histogram Graph"=→"TVE Histogram":T6)  [unwired: 9 in, 4 out]
      n192 = Array Size(array=w38) -> (size(s)=w163:i32)
      n193 = Initialize Array(0.0 ("element"), w137) -> (w135:dbl[])
      n194 = call <vilib>:"Measures of Spread.vi"("type"=w77) -> ("spread value"=→"spread value":dbl)  [unwired: 9 in, 1 out]
      n195 = Initialize Array(0.0 ("element"), w163) -> (w161:dbl[])
      n196 = call "Statistical measure - basics - 3.vi"("Data measured"=w21, "Data reference"=w12) -> ("Statistcs"=w153:T7)  [unwired: 12 in, 1 out]
      n197 = call "Statistical measure - basics - 4.vi"("Data measured"=w61, "Data reference"=w62) -> ("Statistcs"=w150:T7)  [unwired: 12 in, 1 out]
      n198 = call "Statistical measure - basics - 2.vi"("Data measured"=w34, "Data reference"=w135) -> ("Statistcs"=w157:T7)  [unwired: 12 in, 1 out]
      n199 = call "Statistical measure - basics - 1.vi"("Data measured"=w38, "Data reference"=w161) -> ("Statistcs"=w160:T7)  [unwired: 12 in, 1 out]
      n200 = call "Statistical measure - basics percentual - 1.vi"("Data measured"=w30, "Data reference"=w60) -> ("Statistcs"=w166:T7)  [unwired: 12 in, 1 out]
      n201 = Unbundle By Name(w150) -> ("max dev"=w95:dbl, "mean dev"=w152:dbl, "min dev"=w151:dbl)
      n202 = Unbundle By Name(w153) -> ("max dev"=w96:dbl, "mean dev"=w154:dbl, "min dev"=w138:dbl)
      n203 = Unbundle By Name(w157) -> ("max dev"=w97:dbl, "mean dev"=w156:dbl, "min dev"=w155:dbl)
      n204 = Unbundle By Name(w166) -> ("max dev"=w99:dbl, "mean dev"=w165:dbl, "min dev"=w164:dbl)
      n205 = Unbundle By Name(w160) -> ("max dev"=w98:dbl, "mean dev"=w159:dbl, "min dev"=w158:dbl)
      n206 = Build Array(w95, w152, w151) -> (w92:dbl[])
      n207 = Build Array(w96, w154, w138) -> (w93:dbl[])
      n208 = Build Array(w97, w156, w155) -> (w89:dbl[])
      n209 = Build Array(w98, w159, w158) -> (w88:dbl[])
      n210 = Build Array(w99, w165, w164) -> (w94:dbl[])
      n211 = call "Convert to Dynamic Data7"("Array"=w92) -> ("Dynamic Data Type"=w145:dynamicdata)  [unwired: 3 in]
      n212 = call "Convert to Dynamic Data6"("Array"=w93) -> ("Dynamic Data Type"=w146:dynamicdata)  [unwired: 3 in]
      n213 = call "Convert to Dynamic Data4"("Array"=w94) -> ("Dynamic Data Type"=w149:dynamicdata)  [unwired: 3 in]
      n214 = Negate(x=w49) -> (-x=w43:dbl[])
      n215 = Negate(x="busca freq") -> (-x=w47:dbl)
      n216 = call "Convert to Dynamic Data3"("Array"=w89) -> ("Dynamic Data Type"=w148:dynamicdata)  [unwired: 3 in]
      n217 = call "Convert to Dynamic Data5"("Array"=w88) -> ("Dynamic Data Type"=w147:dynamicdata)  [unwired: 3 in]
      n218 = Interpolate 1D Array(1:"frequency 2", 2:w43) -> (0:→"mag correspondente":dbl)
      n219 = Threshold 1D Array(2:w47, 3:w43) -> (0:w52:dbl)  [unwired: 1 in]
      "fractional index" <- w52
      n220 = Multiply(x=w52, y=25.0) -> (x*y=→"x*y":dbl)
      n221 = Merge Signals(w149, w148, w147, w146, w145) -> (w144:dynamicdata)
      n222 = call "Build Table"("Signals"=w144) -> ("Table"=w111:string[][])  [unwired: 4 in, 6 out]
      n223 = Transpose 2D Array(2D array=w111) -> (transposed array=→"Table 2":string[][])
      "ROCOF\nreference" <- w62
      "ROCOF\nmeasured" <- w61
      "Frequency\nreference" <- w12
      "Frequency\nmeasured" <- w21
      "Phase\nreference" <- w78
      "Magnitude\nreference" <- w60
    }
    frame #1 {
      n224 = case shown="\"Frequency reference\"" "X data" {
        tunnel: [w607 w609 w611 w613 w615 w617 w619 w621 w623] -> w563
        tunnel: ["Magnitude (p.u)" "Desvio de magnitude (p.u)" "Fase (°)" "Fase (°)" "Desvio de fase (°)" "Frequência (Hz)" "Frequência (Hz)" "Desvio de frequência (Hz)" "Magnitude (p.u)"] -> w562
        frame "Magnitude measured" {
          n225 = local read "Magnitude\nmeasured"() -> (w607:dbl[])
        }
        frame "Magnitude deviation" {
          n226 = local read "Magnitude deviation"() -> (w609:dbl[])
        }
        frame "Phase reference" {
          n227 = local read "Phase\nreference"() -> (w611:dbl[])
        }
        frame "Phase measured" {
          n228 = local read "Phase\nmeasured"() -> (w613:dbl[])
        }
        frame "Phase deviation" {
          n229 = local read "Phase deviation"() -> (w615:dbl[])
        }
        frame "Frequency reference" {
          n230 = local read "Frequency\nreference"() -> (w617:dbl[])
        }
        frame "Frequency measured" {
          n231 = local read "Frequency\nmeasured"() -> (w619:dbl[])
        }
        frame "Frequency deviation" {
          n232 = local read "Frequency deviation"() -> (w621:dbl[])
        }
        frame "Magnitude reference" {
          n233 = local read "Magnitude\nreference"() -> (w623:dbl[])
        }
      }
      n234 = case shown="\"Magnitude deviation\"" "Y data" {
        tunnel: [w589 w591 w593 w595 w597 w599 w601 w603 w605] -> w556
        tunnel: ["Magnitude (p.u)" "Desvio de magnitude (p.u)" "Fase (°)" "Fase (°)" "Desvio de fase (°)" "Frequência (Hz)" "Frequência (Hz)" "Desvio de frequência (Hz)" "Magnitude (p.u)"] -> w561
        frame "Magnitude measured" {
          n235 = local read "Magnitude\nmeasured"() -> (w589:dbl[])
        }
        frame "Magnitude deviation" {
          n236 = local read "Magnitude deviation"() -> (w591:dbl[])
        }
        frame "Phase reference" {
          n237 = local read "Phase\nreference"() -> (w593:dbl[])
        }
        frame "Phase measured" {
          n238 = local read "Magnitude\nmeasured"() -> (w595:dbl[])
        }
        frame "Phase deviation" {
          n239 = local read "Phase deviation"() -> (w597:dbl[])
        }
        frame "Frequency reference" {
          n240 = local read "Frequency\nreference"() -> (w599:dbl[])
        }
        frame "Frequency measured" {
          n241 = local read "Frequency\nmeasured"() -> (w601:dbl[])
        }
        frame "Frequency deviation" {
          n242 = local read "Frequency deviation"() -> (w603:dbl[])
        }
        frame "Magnitude reference" {
          n243 = local read "Magnitude\nreference"() -> (w605:dbl[])
        }
      }
      n244 = case shown="True" TRUE {
        tunnel: w561 -> [_ w587]
        frame False {
        }
        frame True {
          n245 = control-ref of="Curve fit"() -> (w586:refnum<vi>)
          n246 = control-ref of="Fit deviation"() -> (w585:refnum<vi>)
          n247 = property on="Property Node" class="WFGraph (strict)"(reference=w586, "YScale.NameLbl.Text"=w587) -> ()  [unwired: 1 in, 2 out]
          n248 = property on="Property Node" class="WFGraph (strict)"(reference=w585, "YScale.NameLbl.Text"=w587) -> ()  [unwired: 1 in, 2 out]
        }
      }
      n249 = case shown="\"Sinusoidal\"" "Type" {
        tunnel: w556 -> [w630 w638 w646 w652 _]
        tunnel: w563 -> [w629 w637 w645 w651 _]
        tunnel: [w625 w631 w641 w650 _] -> w558
        tunnel: [w628 w635 w640 w649 w659] -> w557
        tunnel: [w624 w636 w644 w648 _] -> _
        frame "Linear" {
          n250 = call <vilib>:"Linear Fit.vi"("Y"=w630, "X"=w629) -> ("Best Linear Fit"=w628:dbl[], "slope"=w627:dbl, "intercept"=w626:dbl, "residue"=w624:dbl)  [unwired: 9 in, 1 out]
          n251 = Build Array(w627, w626) -> (w625:dbl[])
        }
        frame "Exponencial" {
          n252 = call <vilib>:"Exponential Fit.vi"("Y"=w638, "X"=w637) -> ("Best Exponential Fit"=w635:dbl[], "amplitude"=w634:dbl, "damping"=w633:dbl, "offset"=w632:dbl, "residue"=w636:dbl)  [unwired: 8 in, 1 out]
          n253 = Build Array(w634, w633, w632) -> (w631:dbl[])
        }
        frame "Logarithm" {
          w639 = 2.71828 items=["e"=2.71828, "2"=2.0, "10"=10.0] ("base")
          n254 = call <vilib>:"Logarithm Fit.vi"("Y"=w646, "base"=w639, "X"=w645) -> ("Best Logarithm Fit"=w640:dbl[], "amplitude"=w643:dbl, "scale"=w642:dbl, "residue"=w644:dbl)  [unwired: 8 in, 1 out]
          n255 = Build Array(w643, w642) -> (w641:dbl[])
        }
        frame "Polynomial" {
          n256 = call <vilib>:"General Polynomial Fit.vi"("Y"=w652, "polynomial order"="polynomial order", "X"=w651) -> ("Best Polynomial Fit"=w649:dbl[], "Polynomial Coefficients"=w650:dbl[], "residue"=w648:dbl)  [unwired: 9 in, 1 out]
        }
        frame "Sinusoidal" {
          n257 = Bundle("Numeric"="Numeric", "Numeric"="Numeric") -> (w654:cluster{"Numeric":dbl, "Numeric":dbl})  [unwired: 1 in]
          "output cluster" <- w654
          n258 = call <vilib>:"Sine Waveform.vi"("offset"="offset", "sampling info"=w654, "phase"="phase", "amplitude"="amplitude", "frequency"="frequency") -> ("signal out"=w660:waveform(dbl))  [unwired: 5 in, 1 out]
          n259 = Unbundle By Name(w660) -> ("Y"=w659:dbl[])
        }
      }
      n260 = case shown="False" FALSE {
        tunnel: w563 -> [_ w584]
        tunnel: w562 -> [_ w583]
        tunnel: w558 -> [w570 w573]
        tunnel: w557 -> [w571 w574]
        tunnel: w556 -> [w572 w575]
        tunnel: [w572 w575] -> w567
        tunnel: [w571 w574] -> w568
        tunnel: [w570 w573] -> w569
        frame False {
        }
        frame True {
          n261 = Array Max & Min(array=w584) -> (max value=w578:dbl, min value=w576:dbl)  [unwired: 2 out]
          n262 = Array Size(array=w584) -> (size(s)=w579:i32)
          n263 = Subtract(x=w578, y=w576) -> (x-y=w580:dbl)
          n264 = Divide(x=w580, y=w579) -> (x/y=w577:dbl)
          n265 = control-ref of="Curve fit"() -> (w582:refnum<vi>)
          n266 = control-ref of="Fit deviation"() -> (w581:refnum<vi>)
          n267 = property on="Property Node" class="WFGraph (strict)"(reference=w582, "XScale.NameLbl.Text"=w583, "XScale.Maximum"=w578, "XScale.Minimum"=w576) -> ()  [unwired: 1 in, 2 out]
          n268 = property on="Property Node" class="WFGraph (strict)"(reference=w581, "XScale.NameLbl.Text"=w583, "XScale.Maximum"=w578, "XScale.Minimum"=w576, "XScale.Offset"=w576, "XScale.Multiplier"=w577) -> ()  [unwired: 1 in, 2 out]
        }
      }
      n269 = call "Convert to Dynamic Data12"("Array"=w569) -> ("Dynamic Data Type"=w554:dynamicdata)  [unwired: 3 in]
      n270 = Build Array(w567, w568) -> (→"Curve fit":dbl[][])
      n271 = Subtract(x=w567, y=w568) -> (x-y=w549:dbl[])
      n272 = call "Build Table3"("Signals"=w554) -> ("Table"=w553:string[][])  [unwired: 4 in, 6 out]
      n273 = Multiply(x=w549, y=100) -> (x*y=→"Fit deviation":dbl[])
      n274 = call <vilib>:"Correlation Coefficient.vi"("Y"=w568, "X"=w567) -> ("r^2"=→"R^2":dbl, "correlation coefficient r"=→"Correlation\ncoefficient (R)":dbl)  [unwired: 8 in]
      n275 = Transpose 2D Array(2D array=w553) -> (transposed array=→"Coefficients":string[][])
    }
  }
